vi "End transform.vi"(8 "error in":errorcluster, 10 "End transform":dbl[](array[numeric])) -> (0 "error out":errorcluster)   [LabVIEW 2013]
panel:
  # "When move_to.vi is used \"Pose\" mode, the positions are interpreted as a pose using ZYX Euler angles.  The \"End transform\" can be understood as the null pose of an end-effector (in stage coordinates) .  Then the commanded pose is the desired pose of the end effector."
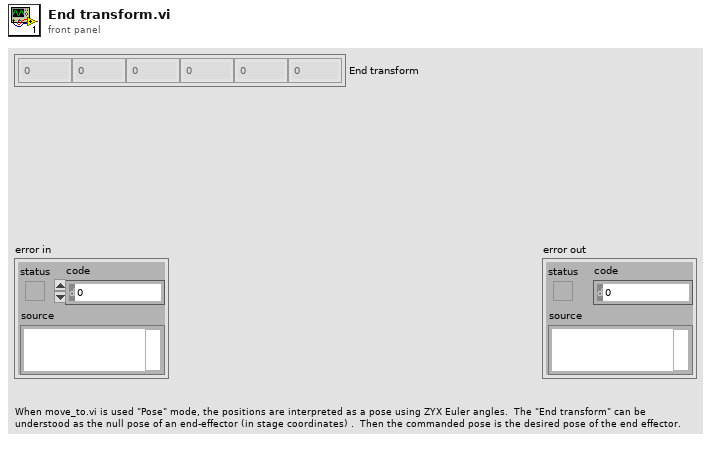
[diagram p1: front panel]
types:
  T1 = typedef "motion_variables.ctl" = cluster{"Motion command":refnum<k21>, "Motion status":refnum<k21>, "Emergency stop":refnum<k21>, "End transform":refnum<k21>, "Home position":refnum<k21>, "Axis offsets":refnum<k21>}
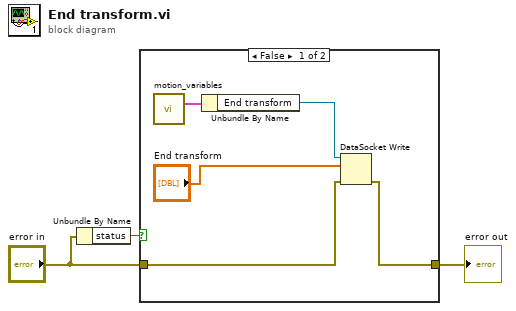
[diagram p0: block diagram]
diagram:
  n1 = Unbundle By Name("error in") -> ("status"=w1:bool)
  n2 = case shown="False" w1 {
    tunnel: [w5 w9] -> w3
    tunnel: "error in" -> [w4 w9]
    frame False {
      n3 = call "motion_variables.vi"() -> ("Motion variables"=w8:T1)  [unwired: 11 in]
      n4 = Unbundle By Name(w8) -> ("End transform"=w7:refnum<k21>)
      n5 = DataSocket Write(8:w4, 10:"End transform", 11:w7) -> (0:w5:errorcluster)  [unwired: 1 in, 2 out]
    }
    frame True {
    }
  }
  "error out" <- w3
